vi "Get Data Source.vi"(8 "error in (no error)":errorcluster, 11 "Sqlite Database Manager in":refnum<class "Sqlite Database Manager.lvclass">) -> (0 "error out":errorcluster, 2 "Data Source":string, 3 "Sqlite Database Manager out":refnum<class "Sqlite Database Manager.lvclass">)   [LabVIEW 2019, in "HierDAL Library.lvlib" / "Database.lvlib" / "Sqlite Database Manager.lvclass"]
uses:
  Sqlite Database Manager.lvclass
  Sqlite Database Manager.lvclass/Sqlite Database Manager.ctl
  System.Data.SQLite
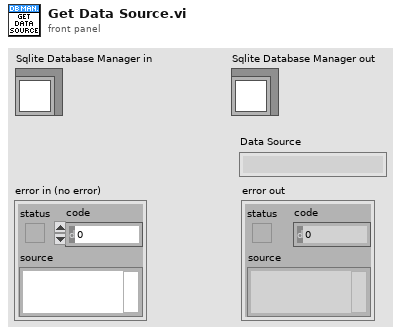
[diagram p1: front panel]
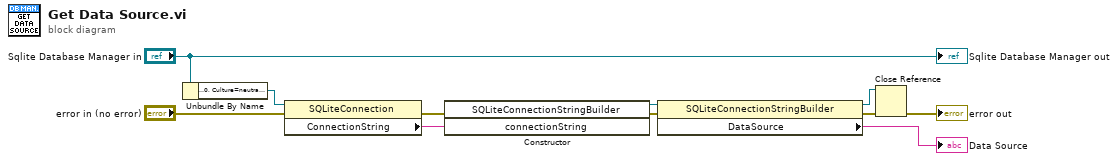
[diagram p0: block diagram]
diagram:
  n1 = Unbundle By Name("Sqlite Database Manager in") -> ("Connection"=w9:refnum<k24>)
  n2 = property class="SQLiteConnection"(reference=w9, error in="error in (no error)") -> (error out=w8:errorcluster, "ConnectionString"=w7:string)  [unwired: 1 out]
  n3 = constructor class="SQLiteConnectionStringBuilder"(error in=w8, "connectionString"=w7) -> (reference out=w5:refnum<k24>, error out=w6:errorcluster)  [unwired: 2 in, 2 out]
  n4 = property class="SQLiteConnectionStringBuilder"(reference=w5, error in=w6) -> (reference out=w3:refnum<k24>, error out=w4:errorcluster, "DataSource"=→"Data Source":string)
  n5 = Close Reference(reference=w3, error in (no error)=w4) -> (error out=→"error out":errorcluster)
  "Sqlite Database Manager out" <- "Sqlite Database Manager in"
